vi "getRfUnits.vi"(8 "error in (no error)":errorcluster, 10 "channel_name":string, 11 "ChannelArray in":refnum<class "ChannelArray.lvclass">) -> (0 "error out":errorcluster, 1 "phase_units":string, 2 "freq_units":string, 3 "ChannelArray out":refnum<class "ChannelArray.lvclass">)   [LabVIEW 2011, in "Tools.lvlib" / "DatabaseHelpers.lvlib" / "ChannelArray.lvclass"]
uses:
  ChannelArray.lvclass
  Channel/RfOutputChannel/RfOutputChannel.lvclass
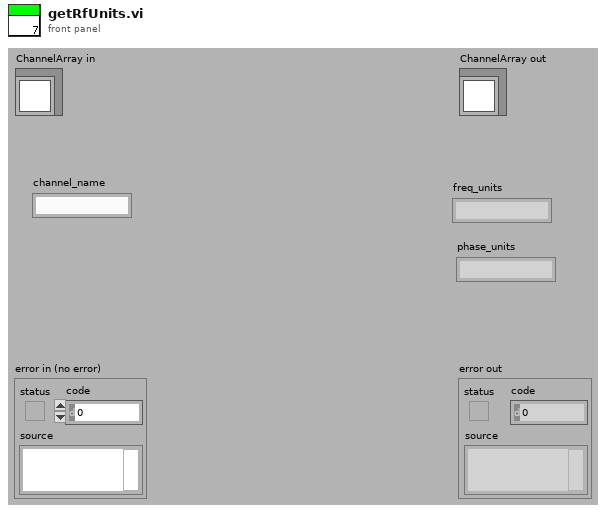
[diagram p1: front panel]
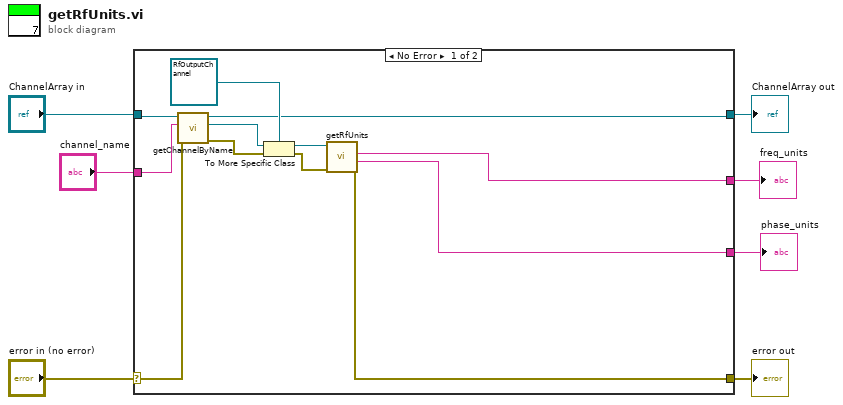
[diagram p0: block diagram]
diagram:
  n1 = case shown="No Error" "error in (no error)" {
    selector: "error in (no error)" -> [w17 w21]
    tunnel: [w8 w21] -> w6
    tunnel: [w11 w20] -> w4
    tunnel: "ChannelArray in" -> [w19 w20]
    tunnel: "channel_name" -> [w18 _]
    tunnel: [w10 _] -> w2
    tunnel: [w9 _] -> w1
    frame No Error {
      n2 = call-dynamic "getChannelByName.vi"("error in (no error)"=w17, "channel_name"=w18, "ChannelArray in"=w19) -> ("error out"=w12:errorcluster, "Channel"=w16:refnum<class "Channel.lvclass">, "ChannelArray out"=w11:refnum<class "ChannelArray.lvclass">)  [unwired: 5 in, 1 out]
      n3 = To More Specific Class(target class=refnum<class "RfOutputChannel.lvclass"> refnum ("RfOutputChannel in"), reference=w16, error in=w12) -> (specific class reference=w14:refnum<class "RfOutputChannel.lvclass">, error out=w13:errorcluster)
      n4 = call "getRfUnits.vi"("error in (no error)"=w13, "RfOutputChannel in"=w14) -> ("error out"=w8:errorcluster, "phase_units"=w9:string, "freq_units"=w10:string)  [unwired: 6 in, 1 out]
    }
    frame Error {
    }
  }
  "error out" <- w6
  "ChannelArray out" <- w4
  "freq_units" <- w2
  "phase_units" <- w1
